vi "SRDG535.set i attribute.vi"(0 "i ref in":refnum<vi>, 2 "i attribute":T1={"GPIB address"="N/A", "Device error"={"status"=FALSE, "code"=0, "source"=""}, "GUI Refs"={"Delete"=refnum, "Device Error"=refnum, "Information"=refnum, "Output"=refnum, "Delay"=refnum, "Trigger"=refnum}, "Output Settings"={"CH T0"={"Inversion"=FALSE, "Amplitude (V)"=1.0, "Offset (V)"=0.0, "Mode"=0, "Load"=FALSE}, "CH A"={"Inversion"=FALSE, "Amplitude (V)"=1.0, "Offset (V)"=0.0, "Mode"=0, "Load"=FALSE}, "CH B"={"Inversion"=FALSE, "Amplitude (V)"=1.0, "Offset (V)"=0.0, "Mode"=0, "Load"=FALSE}, "CH AB"={"Inversion"=FALSE, "Amplitude (V)"=1.0, "Offset (V)"=0.0, "Mode"=0, "Load"=FALSE}, "CH C"={"Inversion"=FALSE, "Amplitude (V)"=1.0, "Offset (V)"=0.0, "Mode"=0, "Load"=FALSE}, "CH D"={"Inversion"=FALSE, "Amplitude (V)"=1.0, "Offset (V)"=0.0, "Mode"=0, "Load"=FALSE}, "CH CD"={"Inversion"=FALSE, "Amplitude (V)"=1.0, "Offset (V)"=0.0, "Mode"=0, "Load"=FALSE}}, "Service ID Rate"=-1, "Service IDs Channelinfo"=[], "Delay Settings"={"CH A"={"rel to"=0, "Delay (s)"=0.0}, "CH B"={"rel to"=0, "Delay (s)"=0.0}, "CH C"={"rel to"=0, "Delay (s)"=0.0}, "CH D"={"rel to"=0, "Delay (s)"=0.0}}, "Trigger Settings"={"trigger"=0, "Impedance"=FALSE, "Slope"=FALSE, "burst count"=2, "external level (V)"=0.0, "Internal/Burst Rate (Hz)"=0.001, "Burst Period"=4}} {"Trigger Settings"."Burst Period" min=4 max=32766; "Trigger Settings"."Internal/Burst Rate (Hz)" min=0.001 max=1000000.0 format="%.3f"; "Trigger Settings"."external level (V)" min=-2.56 max=2.56 format="%.2f"; "Trigger Settings"."burst count" min=2 max=32766; "Trigger Settings"."trigger" scale=0.0..4.0; "Delay Settings"."CH D"."Delay (s)" format="%#_13g"; "Delay Settings"."CH D"."rel to" scale=0.0..3.0; "Delay Settings"."CH C"."Delay (s)" format="%#_13g"; "Delay Settings"."CH C"."rel to" scale=0.0..3.0; "Delay Settings"."CH B"."Delay (s)" format="%#_13g"; "Delay Settings"."CH B"."rel to" scale=0.0..3.0; "Delay Settings"."CH A"."Delay (s)" format="%#_13g"; "Delay Settings"."CH A"."rel to" scale=0.0..3.0; "Output Settings"."CH CD"."Mode" items=["TTL", "NIM", "ECL", "VAR"]; "Output Settings"."CH CD"."Offset (V)" min=-3.0 max=4.0 format="%.2f"; "Output Settings"."CH CD"."Amplitude (V)" min=-3.0 max=4.0 format="%.2f"; "Output Settings"."CH D"."Mode" items=["TTL", "NIM", "ECL", "VAR"]; "Output Settings"."CH D"."Offset (V)" min=-3.0 max=4.0 format="%.2f"; "Output Settings"."CH D"."Amplitude (V)" min=-3.0 max=4.0 format="%.2f"; "Output Settings"."CH C"."Mode" items=["TTL", "NIM", "ECL", "VAR"]; "Output Settings"."CH C"."Offset (V)" min=-3.0 max=4.0 format="%.2f"; "Output Settings"."CH C"."Amplitude (V)" min=-3.0 max=4.0 format="%.2f"; "Output Settings"."CH AB"."Mode" items=["TTL", "NIM", "ECL", "VAR"]; "Output Settings"."CH AB"."Offset (V)" min=-3.0 max=4.0 format="%.2f"; "Output Settings"."CH AB"."Amplitude (V)" min=-3.0 max=4.0 format="%.2f"; "Output Settings"."CH B"."Mode" items=["TTL", "NIM", "ECL", "VAR"]; "Output Settings"."CH B"."Offset (V)" min=-3.0 max=4.0 format="%.2f"; "Output Settings"."CH B"."Amplitude (V)" min=-3.0 max=4.0 format="%.2f"; "Output Settings"."CH A"."Mode" items=["TTL", "NIM", "ECL", "VAR"]; "Output Settings"."CH A"."Offset (V)" min=-3.0 max=4.0 format="%.2f"; "Output Settings"."CH A"."Amplitude (V)" min=-3.0 max=4.0 format="%.2f"; "Output Settings"."CH T0"."Mode" items=["TTL", "NIM", "ECL", "VAR"]; "Output Settings"."CH T0"."Offset (V)" min=-3.0 max=4.0 format="%.2f"; "Output Settings"."CH T0"."Amplitude (V)" min=-3.0 max=4.0 format="%.2f"}, 5 "error in (no error)":errorcluster) -> (14 "i ref out":refnum<vi>, 19 "error out":errorcluster)   [LabVIEW 2014, in "SRDG535.lvlib"]
doc: "Sets the i attribute data of an object.\n\nLicense Agreement for this software:\n\nCopyright (C)\nGesellschaft für Schwerionenforschung, GSI\nPlanckstr. 1\n64291 Darmstadt\nGermany\n\nContact: D.Beck@gsi.de \n\nThis program is free software; you can redistribute it and/or modify it under the terms of the GNU General Public License as published by the Free Software Foundation; either version 2 of the license, or (at your option) any later version.\n\nThis program is distributed in the hope that it will be useful, but WITHOUT ANY WARRANTY; without even the implied warranty of MERCHANTABILITY or FITNESS FOR A PARTICULAR PURPOSE. See the GNU General License for more details (http://www.gnu.org).\n\nGesellschaft für Schwerionenforschung, GSI\nPlanckstr. 1, 64291 Darmstadt, Germany\nFor all questions and ideas contact: M.Richter@gsi.de, H.Brand@gsi.de or D.Beck@gsi.de.\nLast update: 17-JUN-2004"
uses:
  SRDG535.lvlib
  SRDG535.i attribute.ctl
  SRDG535.Output.ctl
  SRDG535.Channel Output.ctl
  SRDG535.Delay.ctl
  SRDG535.Trigger.ctl
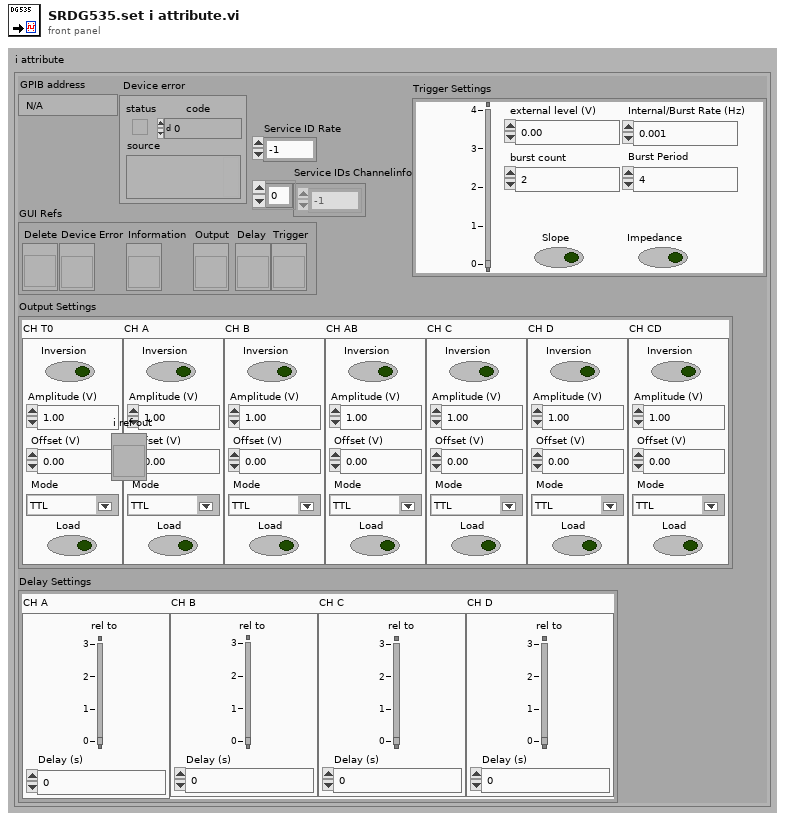
[diagram p1: front panel]
types:
  T1 = typedef "SRDG535.lvlib/SRDG535.i attribute.ctl" = cluster{"GPIB address":string, "Device error":errorcluster, "GUI Refs":cluster{"Delete":refnum<vi>, "Device Error":refnum<vi>, "Information":refnum<vi>, "Output":refnum<vi>, "Delay":refnum<vi>, "Trigger":refnum<vi>}, "Output Settings":T2, "Service ID Rate":i32, "Service IDs Channelinfo":i32[], "Delay Settings":T4, "Trigger Settings":T5}
  T2 = typedef "SRDG535.lvlib/SRDG535.Output.ctl" = cluster{"CH T0":T3, "CH A":T3, "CH B":T3, "CH AB":T3, "CH C":T3, "CH D":T3, "CH CD":T3}
  T3 = typedef "SRDG535.lvlib/SRDG535.Channel Output.ctl" = cluster{"Inversion":bool, "Amplitude (V)":dbl, "Offset (V)":dbl, "Mode":i32, "Load":bool}
  T4 = typedef "SRDG535.lvlib/SRDG535.Delay.ctl" = cluster{"CH A":cluster{"rel to":u32, "Delay (s)":dbl}, "CH B":cluster{"rel to":u32, "Delay (s)":dbl}, "CH C":cluster{"rel to":u32, "Delay (s)":dbl}, "CH D":cluster{"rel to":u32, "Delay (s)":dbl}}
  T5 = typedef "SRDG535.lvlib/SRDG535.Trigger.ctl" = cluster{"trigger":u32, "Impedance":bool, "Slope":bool, "burst count":i32, "external level (V)":sgl, "Internal/Burst Rate (Hz)":dbl, "Burst Period":i32}
  T6 = enum16{"SetAttribute", "GetAttribute", "CreateAttribute", "DestroyAttribute", "DestroyAllAtributes"}
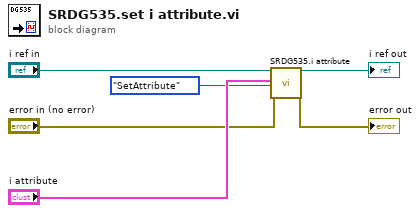
[diagram p0: block diagram]
diagram:
  n1 = call "SRDG535.i attribute.vi"("VI Refnum"="i ref in", "CLASS.i attribute"="i attribute", "Action"=T6."SetAttribute", "error in (no error)"="error in (no error)") -> ("VI Refnum out"=→"i ref out":refnum<vi>, "error out"=→"error out":errorcluster)  [unwired: 13 in, 1 out]
